vi "CheckErrors_Benchmark.vi"() -> ()   [LabVIEW 2017]
uses:
  SoftmotionClass/SoftmotionAxis/SoftmotionAxis.lvclass
  Utilities/StateMachine.ctl
  <vilib>/NI_Real-Time Target Support.lvlib
  Utilities/WordManipulationLibrary.lvlib
panel:
  out "Array":T1[](array[typedef])
  out "appended array":dbl[](array[numeric])
  out "SoftmotionAxis out":refnum<class "SoftmotionAxis.lvclass">
  out "Mean time (us)":dbl format="%.3g"
  in  "Warmup iterations":i32=10
  in  "Calibrate?":bool
  out "Execution histogram":T2(graph)
  out "Standard deviation (us)":dbl format="%.3g"
  out "Max jitter (us)":dbl format="%.3g"
  out "Execution times (us)":dbl[](graph)
  in  "Iterations":i32=1000
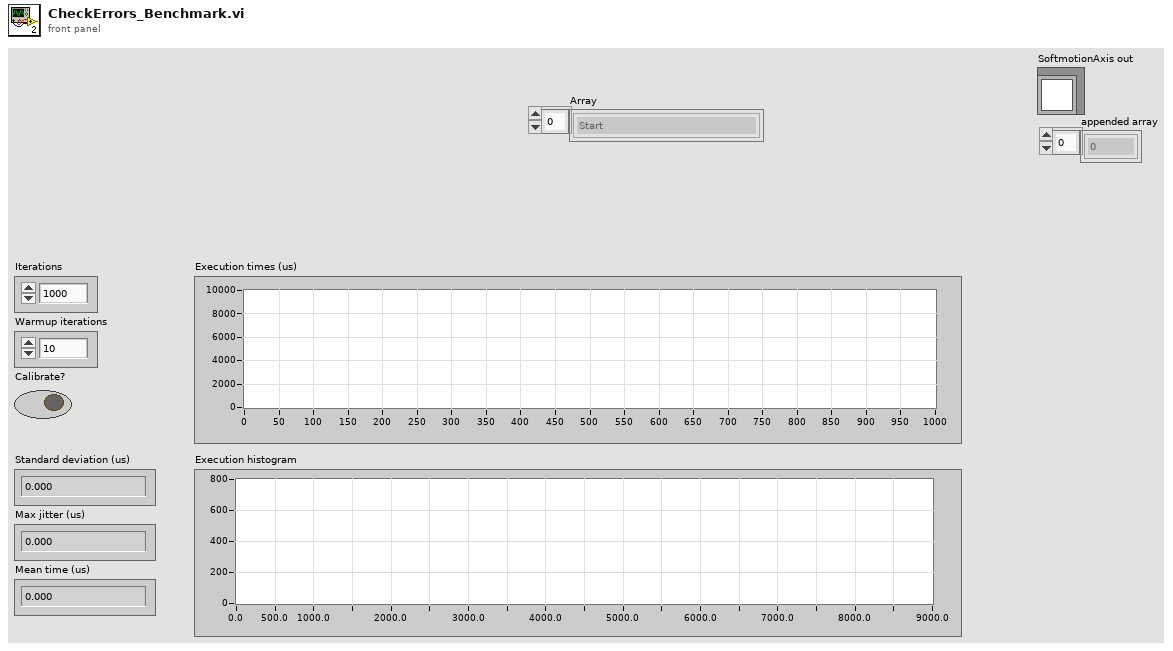
[diagram p1: front panel]
types:
  T1 = typedef "WordManipulationLibrary.lvlib/StateMachine.ctl" = enum16{"Start", "Not Ready to Switch On", "Switch On Disabled", "Ready to Switch On", "Switched On", "Operation enable", "Quick Stop Active", "Fault Reaction Active", "Fault"}
  T2 = cluster{"X Values":dbl[], "Histogram: h(x)":i32[]}
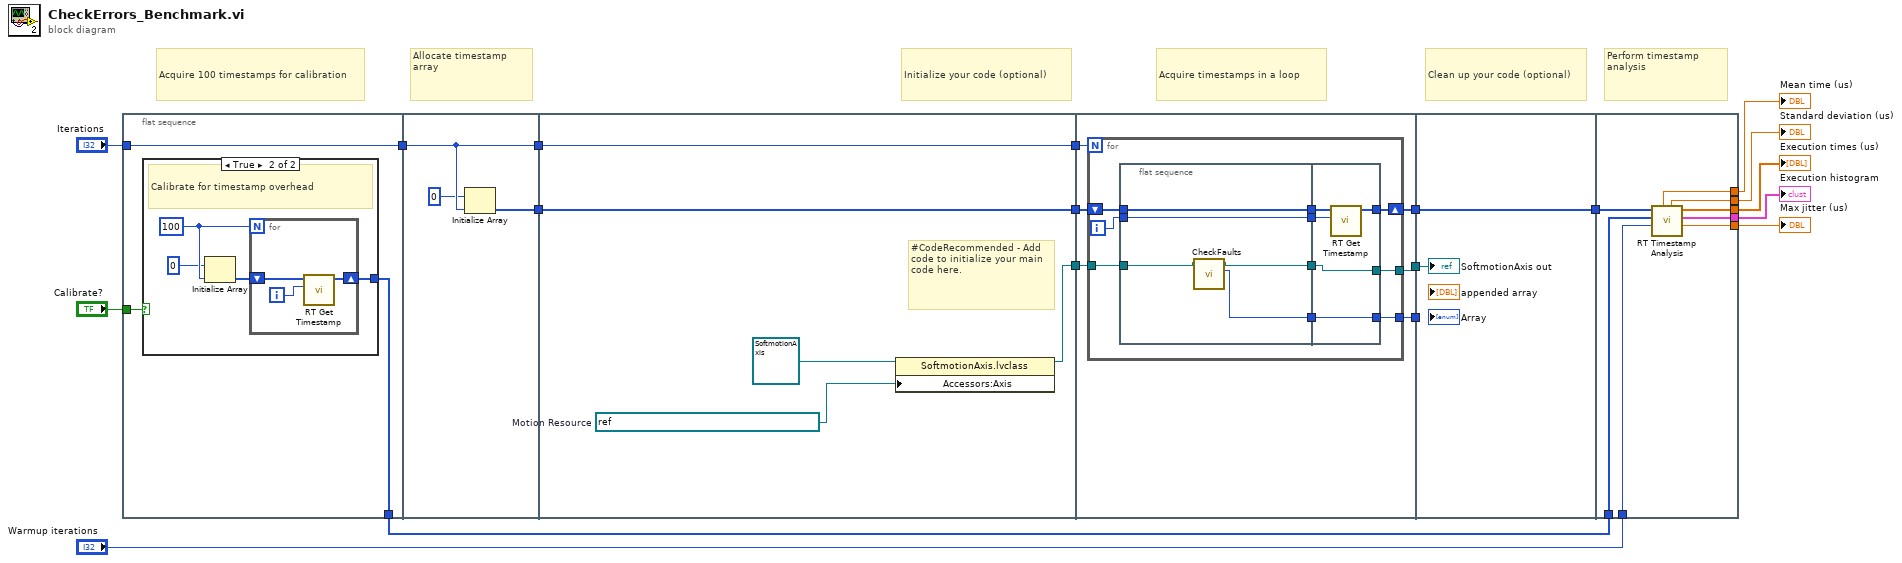
[diagram p0: block diagram]
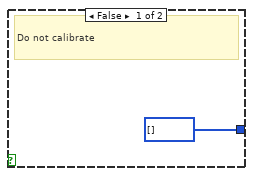
[diagram p2: hidden frame]
diagram:
  # "Perform timestamp analysis"
  # "Clean up your code (optional)"
  # "Acquire timestamps in a loop"
  # "Initialize your code (optional)"
  # "Allocate timestamp array"
  # "Acquire 100 timestamps for calibration"
  n1 = flat-sequence {
    tunnel: "Iterations" -> [w22]
    tunnel: [w22] -> w19
    tunnel: "Calibrate?" -> [w21]
    tunnel: [w20] -> w10
    tunnel: [w32] -> w18
    tunnel: [w33] -> w17
    tunnel: w19 -> [w32]
    tunnel: [w38] -> w16
    tunnel: [w37] -> w15
    tunnel: w18 -> [w38]
    tunnel: w17 -> [w37]
    tunnel: [w34] -> w3
    tunnel: [w44] -> w14
    tunnel: w16 -> [w43]
    tunnel: w15 -> [w42]
    tunnel: w3 -> [w41]
    tunnel: [w40] -> w2
    tunnel: [w39] -> w1
    tunnel: w14 -> [w66]
    tunnel: [w66] -> w13
    tunnel: w2 -> [w65]
    tunnel: w1 -> [_]
    tunnel: w13 -> [w74]
    tunnel: w10 -> [w73]
    tunnel: [w72] -> w4
    tunnel: [w71] -> w8
    tunnel: [w70] -> w7
    tunnel: [w69] -> w9
    tunnel: "Warmup iterations" -> [w68]
    tunnel: [w67] -> w5
    frame #0 {
      n2 = case shown="True" w21 {
        tunnel: [u64[] [] w27] -> w20
        frame False {
          # "Do not calibrate"
        }
        frame True {
          w25 = 100
          # "Calibrate for timestamp overhead"
          n3 = Initialize Array(u64 0, w25) -> (w26:u64[])
          n4 = for {
            N: w25 -> [_]
            shift-right: [w28] -> w27
            shift-left: w26 -> [w29]
            i -> [w30]
            n5 = call <vilib>:"RT Get Timestamp.vi"("iteration"=w30, "timestamp array in"=w29) -> ("timestamp array out"=w28:u64[])  [unwired: 1 in, 8 out]
          }
        }
      }
    }
    frame #1 {
      n6 = Initialize Array(u64 0, w32) -> (w33:u64[])
    }
    frame #2 {
      w35 = refnum<k21> "nism://RT CompactRIO Target/Axis 1"  # Motion Resource
      # "#CodeRecommended - Add code to initialize your main code here."
      n7 = property class="SoftmotionAxis.lvclass"(reference=refnum<class "SoftmotionAxis.lvclass"> refnum ("SoftmotionAxis.lvclass"), "Accessors:Axis"=w35) -> (reference out=w34:refnum<class "SoftmotionAxis.lvclass">)  [unwired: 1 in, 1 out]
    }
    frame #3 {
      n8 = for {
        N: w43 -> [_]
        shift-right: [w54] -> w44
        shift-left: w42 -> [w53]
        tunnel: w41 -> [w49]
        tunnel: [w48] -> w40
        tunnel: [w46] -> w39
        i -> [w52]
        n9 = flat-sequence {
          tunnel: w53 -> [w59]
          tunnel: [w59] -> w51
          tunnel: w52 -> [w58]
          tunnel: [w58] -> w50
          tunnel: w49 -> [w57]
          tunnel: [w56] -> w47
          tunnel: [w55] -> w45
          tunnel: [w64] -> w54
          tunnel: w51 -> [w62]
          tunnel: w50 -> [w63]
          tunnel: [w61] -> w48
          tunnel: w47 -> [w61]
          tunnel: [w60] -> w46
          tunnel: w45 -> [w60]
          frame #0 {
            n10 = call "CheckFaults.vi"("SoftmotionAxis in"=w57) -> ("State Out"=w55:T1, "SoftmotionAxis out"=w56:refnum<class "SoftmotionAxis.lvclass">)  [unwired: 8 in, 1 out]
          }
          frame #1 {
            n11 = call <vilib>:"RT Get Timestamp.vi"("iteration"=w63, "timestamp array in"=w62) -> ("timestamp array out"=w64:u64[])  [unwired: 1 in, 8 out]
          }
        }
      }
    }
    frame #4 {
      "SoftmotionAxis out" <- w65
    }
    frame #5 {
      n12 = call <vilib>:"RT Timestamp Analysis.vi"("warmup iterations"=w68, "calibration array"=w73, "timestamp array"=w74) -> ("max jitter (uS)"=w71:dbl, "execution histogram"=w72:T2, "execution times (uS)"=w69:dbl[], "standard deviation (uS)"=w70:dbl, "mean time (uS)"=w67:dbl)  [unwired: 1 in, 3 out]
    }
  }
  "Execution times (us)" <- w9
  "Max jitter (us)" <- w8
  "Standard deviation (us)" <- w7
  "Execution histogram" <- w4
  "Mean time (us)" <- w5
